vi "Rotate Initial Array.vi"(11 "Array in":u32[][](array[numeric])) -> (3 "Array out":u32[][](array[numeric]))   [LabVIEW 2017, in "Game Engine.lvlib" / "Game Engine.lvclass"]
uses:
  Game Engine.lvclass
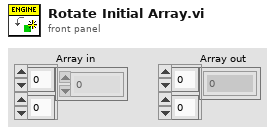
[diagram p1: front panel]
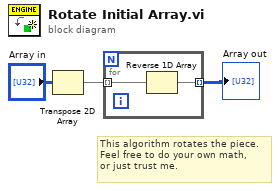
[diagram p0: block diagram]
diagram:
  # "This algorithm rotates the piece.\nFeel free to do your own math,\nor just trust me."
  n1 = Transpose 2D Array(2D array="Array in") -> (transposed array=w1:u32[][])
  n2 = for {
    tunnel: w1 -> [w5] mode=indexing
    tunnel: [w4] -> w3 mode=indexing
    n3 = Reverse 1D Array(array=w5) -> (reversed array=w4:u32[])
  }
  "Array out" <- w3
